vi "printDirectory.vi"(8 "Error In":errorcluster, 10 "nested level":u8, 11 "file":refnum<class "File.lvclass">) -> (0 "Error Out":errorcluster)   [LabVIEW 2014, in "LabVIEW Universal Transcriptor SD Card Library.lvlib"]
uses:
  LabVIEW Universal Transcriptor SD Card Library.lvlib
  File.lvclass
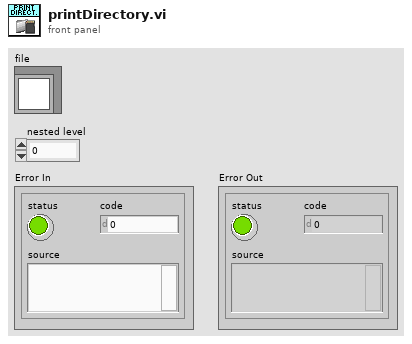
[diagram p1: front panel]
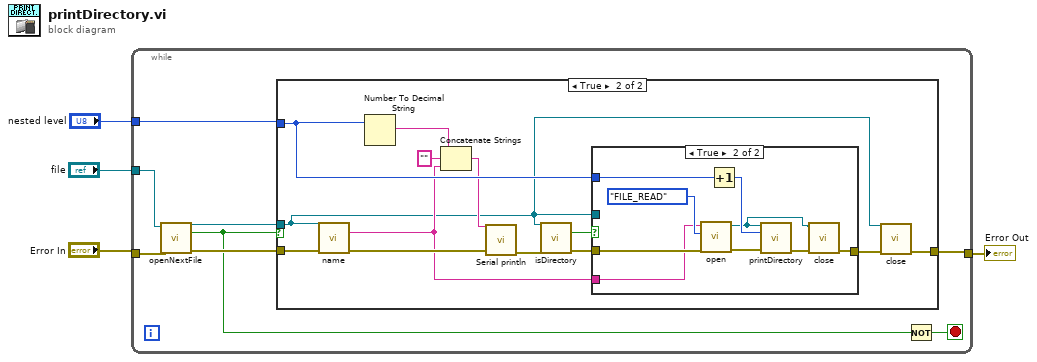
[diagram p0: block diagram]
diagram:
  n1 = while {
    tunnel: "nested level" -> [w9]
    tunnel: "Error In" -> [w6]
    tunnel: [w10] -> w3
    tunnel: "file" -> [w5]
    stop <- w8 stop-if-true
    n2 = call "openNextFile.vi"("error in (no error)"=w6, "File in"=w5) -> ("error out"=w11:errorcluster, "success?"=w7:bool, "File out"=w12:refnum<class "File.lvclass">)  [unwired: 7 in]
    n3 = case shown="True" w7 {
      tunnel: w12 -> [_ w14]
      tunnel: w11 -> [w13 w26]
      tunnel: [w13 w16] -> w10
      tunnel: w9 -> [_ w21]
      frame False {
      }
      frame True {
        n4 = call-dynamic "name.vi"("error in (no error)"=w26, "File in"=w14) -> ("error out"=w25:errorcluster, "file name"=w15:string)  [unwired: 8 in]
        n5 = Number To Decimal String(number=w21) -> (decimal integer string=w20:string)  [unwired: 1 in]
        n6 = Concatenate Strings(w20, "" ("string"), w15) -> (w18:string)
        n7 = call <vilib>:"Serial println.vi"("Error In"=w25, "string in"=w18) -> ("Error Out"=w24:errorcluster)  [unwired: 9 in]
        n8 = call-dynamic "isDirectory.vi"("error in (no error)"=w24, "File in"=w14) -> ("error out"=w23:errorcluster, "is directory?"=w22:bool)  [unwired: 8 in]
        n9 = case shown="True" w22 {
          tunnel: w23 -> [w27 w33]
          tunnel: [w27 w31] -> w17
          tunnel: w14 -> [_ _]
          tunnel: w21 -> [_ w36]
          tunnel: w15 -> [_ w28]
          frame False {
          }
          frame True {
            n10 = call "open.vi"("Error In"=w33, "mode"=enum16{"FILE_READ", "FILE_WRITE"}."FILE_READ", "filepath"=w28) -> ("Error Out"=w32:errorcluster, "File out"=w29:refnum<class "File.lvclass">)  [unwired: 6 in, 1 out]
            n11 = Increment(x=w36) -> (x+1=w35:u8)
            n12 = call "printDirectory.vi"("Error In"=w32, "nested level"=w35, "file"=w29) -> ("Error Out"=w30:errorcluster)  [unwired: 8 in]
            n13 = call-dynamic "close.vi"("error in (no error)"=w30, "File in"=w29) -> ("error out"=w31:errorcluster)  [unwired: 9 in]
          }
        }
        n14 = call-dynamic "close.vi"("error in (no error)"=w17, "File in"=w14) -> ("error out"=w16:errorcluster)  [unwired: 9 in]
      }
    }
    n15 = Not(x=w7) -> (.not. x?=w8:bool)
  }
  "Error Out" <- w3
